vi "Build Waveform Settings.vi"(8 "error in":errorcluster, 10 "Waveform Settings":T1 {"DataType" items=["Double", "ComplexDouble"]}) -> (0 "error out":errorcluster, 2 "Waveform Settings Table":string[][](array[string]))   [LabVIEW 2026]
uses:
  Types/WaveformSettings.ctl
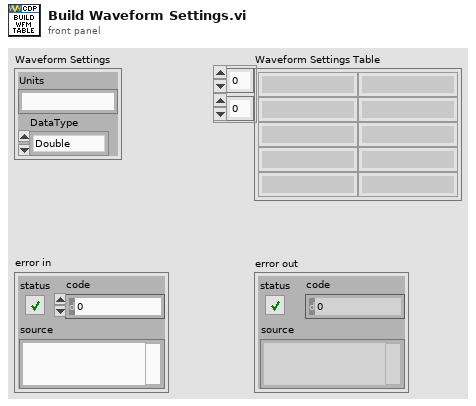
[diagram p1: front panel]
types:
  T1 = typedef "WaveformSettings.ctl" = cluster{"Units":string, "DataType":i32}
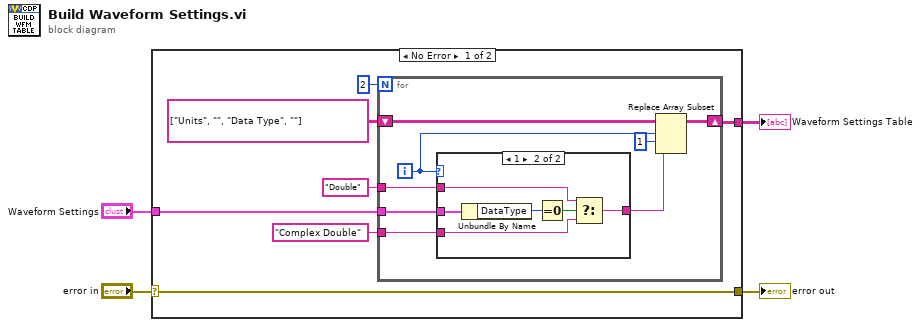
[diagram p0: block diagram]
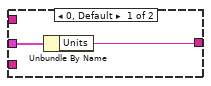
[diagram p2: hidden frame]
diagram:
  n1 = case shown="No Error" "error in" {
    selector: "error in" -> [w5 w28]
    tunnel: "Waveform Settings" -> [w11 _]
    tunnel: [w6 _] -> w3
    tunnel: [w5 w28] -> w1
    frame No Error {
      n2 = for {
        N: 2 -> [_]
        tunnel: w11 -> [w19]
        shift-right: [w17] -> w6
        shift-left: string[][] [["Units", ""], ["Data Type", ""]] -> [w18]
        tunnel: "Double" -> [w16]
        tunnel: "Complex Double" -> [w15]
        i -> [w13]
        n3 = case shown="1" w13 {
          tunnel: w19 -> [w21 w27]
          tunnel: w16 -> [_ w24]
          tunnel: w15 -> [_ w23]
          tunnel: [w20 w22] -> w14
          frame 0, Default {
            n4 = Unbundle By Name(w21) -> ("Units"=w20:string)
          }
          frame 1 {
            n5 = Unbundle By Name(w27) -> ("DataType"=w26:i32)
            n6 = Equal To 0?(x=w26) -> (x = 0?=w25:bool)
            n7 = Select(t=w24, s=w25, f=w23) -> (s? t:f=w22:string)
          }
        }
        n8 = Replace Array Subset(array=w18, new element=w14, index (row)=w13, index (col)=1 ("disabled index (col)")) -> (w17:string[][])
      }
    }
    frame Error {
    }
  }
  "Waveform Settings Table" <- w3
  "error out" <- w1
